vi "Pfeiffer-RVC300.constructor.vi"(0 "name":string, 2 "data in":string, 5 "error in(no error)":errorcluster) -> (14 "i ref out":refnum<vi>, 16 "data out":string, 19 "error out":errorcluster)   [LabVIEW 2014, in "Pfeiffer-RVC300.lvlib"]
doc: "This is the constructor of a class.\n\nLicense Agreement for this software:\n\nCopyright (C)\nMax-Planck-Institut für Kernphysik\nSaupfercheckweg 1\n69117 Heidelberg\nGermany\n\nContact: christopher.borgmann@mpi-hd.mpg.de\n\nThis program is free software: you can redistribute it and/or modify \nit under the terms of the GNU General Public License as published by\nthe Free Software Foundation, either version 3 of the License, or\n(at your option) any later version.\n\nThis program is distributed in the hope that it will be useful,\nbut WITHOUT ANY WARRANTY; without even the implied warranty of\nMERCHANTABILITY or FITNESS FOR A PARTICULAR PURPOSE. See the\nGNU General Public License for more details.\n\nYou should have received a copy of the GNU General Public License\nalong with this program. If not, see <http://www.gnu.org/licenses/>.\n\nMax-Planck-Institut für Kernphysik\nSaupfercheckweg 1, 69117 Heidelberg, Germany\nFor all questions and ideas contact: christopher.borgmann@mpi-hd.mpg.de\nLast update: 08.07.2010"
uses:
  Pfeiffer-RVC300.lvlib
  CS_Core/CSApplicationBaseClasses/DeviceBase/DeviceBase.lvlib
  CS_Core/CSSystem/CSSystemLib/CSSystemLib.lvlib
  CS_Core/CSApplicationBaseClasses/DeviceBase/DeviceBase.myEventNames.ctl
  Pfeiffer-RVC300.i attribute.ctl
  Pfeiffer-RVC300.regulation mode.ctl
  Pfeiffer-RVC300.parameters.ctl
panel:
  in  "attributeType":T1
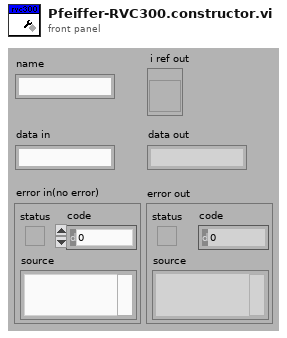
[diagram p1: front panel]
types:
  T1 = typedef "Pfeiffer-RVC300.lvlib/Pfeiffer-RVC300.i attribute.ctl" = cluster{"interfaceInitialized":bool, "VISAResource":refnum<visa-resource-name>, "WaitingTime":u32, "nomValues":T2, "actValues":T2}
  T2 = typedef "Pfeiffer-RVC300.lvlib/Pfeiffer-RVC300.parameters.ctl" = cluster{"regulationMode":T3, "valveType":string, "sensorType":string, "valveState":string, "flow":dbl, "pressure":dbl, "serviceIDs":cluster{"regulationModeID":i32, "valveTypeID":i32, "sensorTypeID":i32, "valveStateID":i32, "flowID":i32, "pressureID":i32}}
  T3 = typedef "Pfeiffer-RVC300.lvlib/Pfeiffer-RVC300.regulation mode.ctl" = enum16{"unknown", "Pressure", "Flow", "Wait"}
  T4 = enum16{"SetAttribute", "GetAttribute", "CreateAttribute", "DestroyAttribute", "DestroyAllAtributes"}
  T5 = typedef "DeviceBase.lvlib/DeviceBase.myEventNames.ctl" = enum16{"lvmsg://Initialize", "lvmsg://Close", "lvmsg://Configure", "lvmsg://Reset", "lvmsg://IDQuery"}
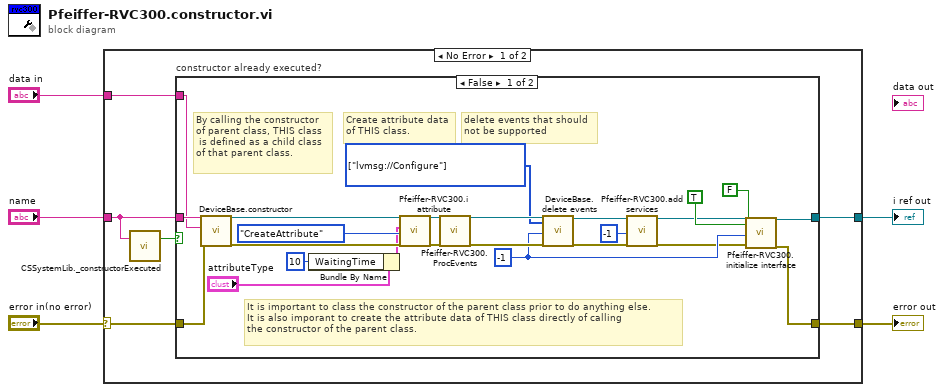
[diagram p0: block diagram]
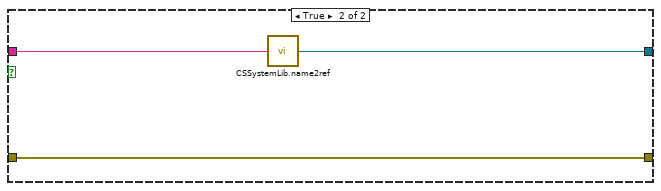
[diagram p2: hidden frame]
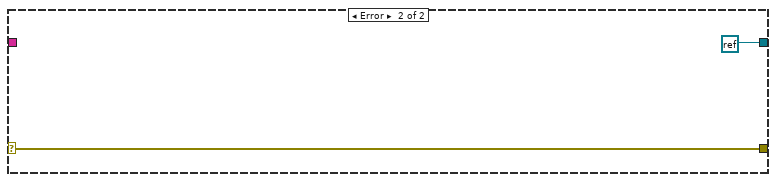
[diagram p3: hidden frame]
diagram:
  n1 = case shown="No Error" "error in(no error)" {
    selector: "error in(no error)" -> [w9 w39]
    tunnel: "name" -> [w8 _]
    tunnel: [w11 refnum<k0> refnum] -> w4
    tunnel: [w10 w39] -> w3
    tunnel: "data in" -> [w6 _]
    frame No Error {
      n2 = call "CSSystemLib._constructorExecuted.vi"("name"=w8) -> ("constructor executed?"=w7:bool)  [unwired: 18 in]
      n3 = case "constructor already executed?" shown="False" w7 {
        tunnel: w8 -> [w33 w38]
        tunnel: [w24 w37] -> w11
        tunnel: [w23 w36] -> w10
        tunnel: w9 -> [w30 w36]
        tunnel: w6 -> [w29 _]
        frame False {
          w26 = T5[] [enum."lvmsg://Configure"] items=["lvmsg://Initialize", "lvmsg://Close", "lvmsg://Configure", "lvmsg://Reset", "lvmsg://IDQuery"] ("events")
          w25 = -1 ("ms timeout (10000)")
          # "delete events that should\nnot be supported"
          # "It is important to class the constructor of the parent class prior to do anything else.\nIt is also imporant to create the attribute data of THIS class directly of calling\nthe constructor of the parent class."
          # "Create attribute data\nof THIS class."
          # "By calling the constructor\nof parent class, THIS class\n is defined as a child class\nof that parent class."
          n4 = call "DeviceBase.constructor.vi"("name"=w33, "data in"=w29, "error in (no error)"=w30) -> ("i ref out"=w35:refnum<vi>, "error out"=w34:errorcluster)  [unwired: 14 in, 1 out]
          n5 = Bundle By Name(cluster="attributeType", "WaitingTime"=u32 10) -> (w19:T1)
          n6 = call "Pfeiffer-RVC300.i attribute.vi"("VI Refnum"=w35, "CLASS.i attribute"=w19, "Action"=T4."CreateAttribute", "error in (no error)"=w34) -> ("VI Refnum out"=w32:refnum<vi>, "error out"=w31:errorcluster)  [unwired: 13 in, 1 out]
          n7 = call "Pfeiffer-RVC300.ProcEvents.vi"("i ref in"=w32, "error in"=w31) -> ("i ref out"=w28:refnum<vi>, "error out"=w27:errorcluster)  [unwired: 16 in]
          n8 = call "DeviceBase.delete events.vi"("i ref in"=w28, "events"=w26, "ms timeout (10000)"=w25, "error in (no error)"=w27) -> ("i ref out"=w16:refnum<vi>, "error out"=w14:errorcluster)  [unwired: 13 in, 1 out]
          n9 = call "Pfeiffer-RVC300.add services.vi"("i ref in"=w16, "ms timeout (10000)"=-1, "error in (no error)"=w14) -> ("i ref out"=w15:refnum<vi>, "error out"=w13:errorcluster)  [unwired: 14 in, 1 out]
          n10 = call "Pfeiffer-RVC300.initialize interface.vi"("i ref in"=w15, "queryID"=TRUE, "resetDevice"=FALSE, "ms timeout (10000)"=w25, "error in (no error)"=w13) -> ("i ref out"=w24:refnum<vi>, "error out"=w23:errorcluster)  [unwired: 11 in, 2 out]
        }
        frame True {
          n11 = call "CSSystemLib.name2ref.vi"("name"=w38) -> ("obj refnum"=w37:refnum<vi>)
        }
      }
    }
    frame Error {
    }
  }
  "i ref out" <- w4
  "error out" <- w3
